vi "Event Create Once.vi"() -> (3 "Camera Events":refnum<user-event>, 4 "Camera Events 2":T1={"Event Type"=enum."Set White Balance", "Setpoint"=100, "Camera"="HD USB Camera "})   [LabVIEW 2019]
uses:
  Camera Set Up/Camera Event Cluster.ctl
  Camera Set Up/Event Setup Types.ctl
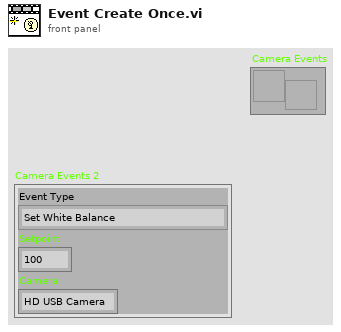
[diagram p1: front panel]
types:
  T1 = typedef "Camera Event Cluster.ctl" = cluster{"Event Type":T2, "Setpoint":i64, "Camera":string}
  T2 = typedef "Event Setup Types.ctl" = enum16{"Save Data", "Set White Balance", "Set Brightness", "Set Exposure", "Update Brightness", "Update Exposure", "Update White Balance", "Exit"}
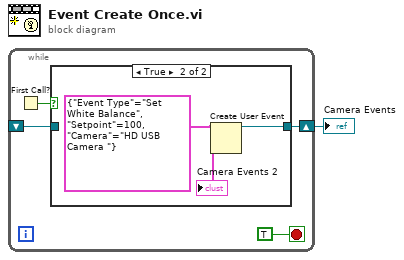
[diagram p0: block diagram]
diagram:
  n1 = while {
    shift-right: [w3] -> w1
    shift-left: _ -> [w2]
    stop <- TRUE stop-if-true
    n2 = First Call?() -> (First Call?: T/F=w4:bool)
    n3 = case shown="True" w4 {
      tunnel: [w6 w8] -> w3
      tunnel: w2 -> [w6 _]
      frame False {
      }
      frame True {
        w7 = T1 {"Event Type"=enum."Set White Balance", "Setpoint"=100, "Camera"="HD USB Camera "} ("Camera Events")
        n4 = Create User Event(user event datatype=w7) -> (user event=w8:refnum<user-event>)  [unwired: 1 in, 1 out]
        "Camera Events 2" <- w7
      }
    }
  }
  "Camera Events" <- w1
